vi "CheckPosition.vi"(11 "Accelerometr data":T1) -> (3 "State":string)   [LabVIEW 2015]
uses:
  ctrls/AccelerometerData.ctl
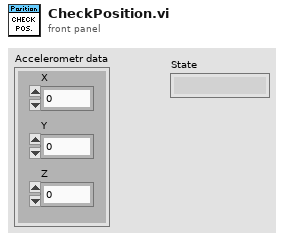
[diagram p1: front panel]
types:
  T1 = typedef "AccelerometerData.ctl" = cluster{"X":dbl, "Y":dbl, "Z":dbl}
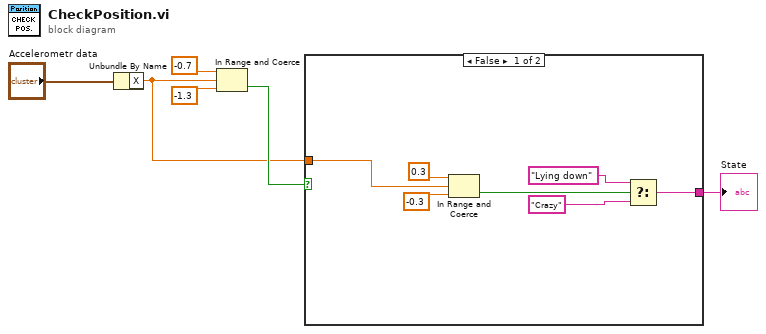
[diagram p0: block diagram]
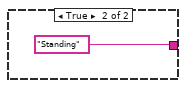
[diagram p2: hidden frame]
diagram:
  n1 = Unbundle By Name("Accelerometr data") -> ("X"=w2:dbl)
  n2 = In Range and Coerce(upper limit=-0.7, x=w2, lower limit=-1.3 ("upper limit")) -> (In Range?=w3:bool)  [unwired: 1 out]
  n3 = case shown="False" w3 {
    tunnel: [w8 "Standing"] -> w1
    tunnel: w2 -> [w11 _]
    frame False {
      n4 = In Range and Coerce(upper limit=0.3, x=w11, lower limit=-0.3 ("upper limit")) -> (In Range?=w10:bool)  [unwired: 1 out]
      n5 = Select(t="Lying down", s=w10, f="Crazy") -> (s? t:f=w8:string)
    }
    frame True {
    }
  }
  "State" <- w1
